vi "Constructor_FastTreeView.vi"(7 "FastTreeView in":refnum<class "FastTreeView.lvclass">, 8 "error in (no error)":errorcluster, 10 "LvTreeGrid":refnum<k24>) -> (0 "error out":errorcluster, 3 "FastTreeView out":refnum<class "FastTreeView.lvclass">)   [LabVIEW 2025, in "FastTreeView.lvclass"]
uses:
  FastTreeView.lvclass
  C:/Git/FastTreeView/FastTreeView/LV/FastTreeView/dll/FastTreeView.dll
  dll/FastTreeView.dll
  FastTreeView.lvclass/FastTreeView.ctl
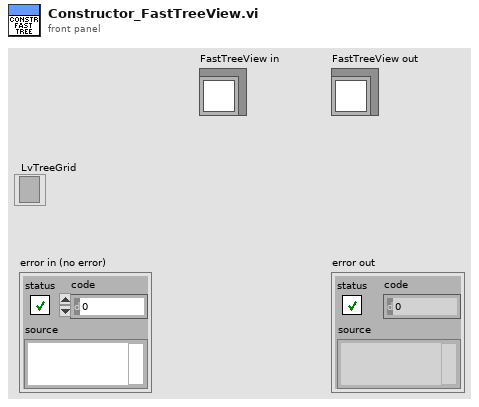
[diagram p1: front panel]
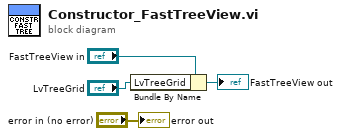
[diagram p0: block diagram]
diagram:
  n1 = Bundle By Name(cluster="FastTreeView in", "LvTreeGrid"="LvTreeGrid") -> (→"FastTreeView out":refnum<class "FastTreeView.lvclass">)
  "error out" <- "error in (no error)"
